vi "Pause.vi"(8 "error in (no error)":errorcluster, 11 "Pause-Resume":refnum<vi>) -> (0 "error out":errorcluster)   [LabVIEW 2014]
panel:
  # "LICENSED MATERIALS – PROPERTY OF IBM\nCopyright IBM Corp. 2016,\nALL RIGHTS RESERVED"
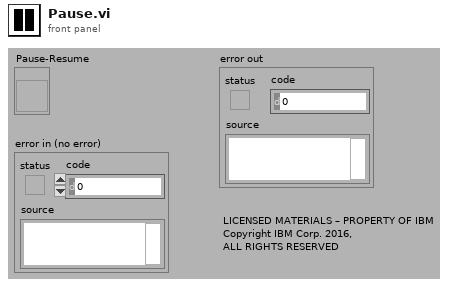
[diagram p1: front panel]
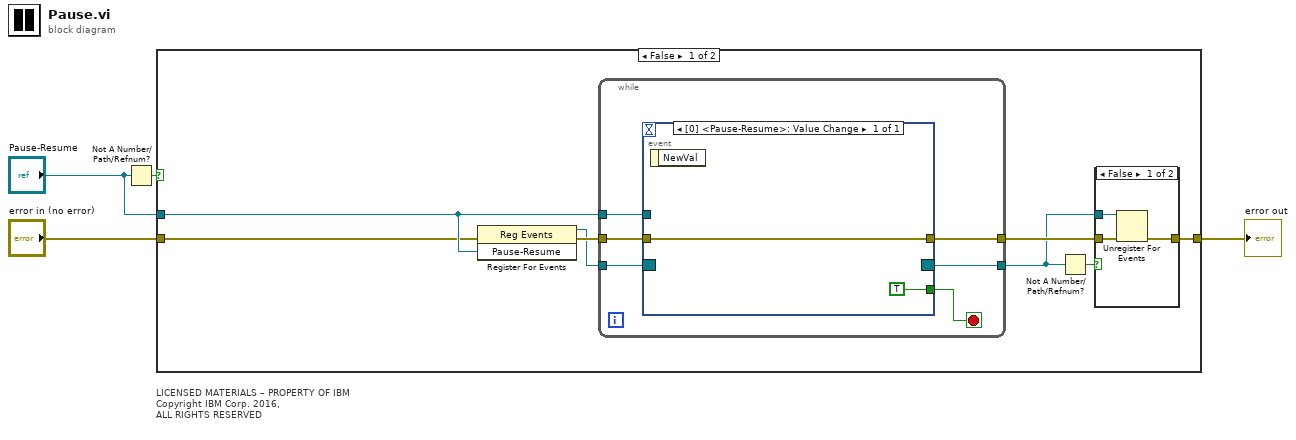
[diagram p0: block diagram]
diagram:
  # "LICENSED MATERIALS – PROPERTY OF IBM\nCopyright IBM Corp. 2016,\nALL RIGHTS RESERVED"
  n1 = Not A Number/Path/Refnum?(number/path/refnum="Pause-Resume") -> (NaN/Path/Refnum?=w3:bool)
  n2 = case shown="False" w3 {
    tunnel: "error in (no error)" -> [w5 w25]
    tunnel: [w9 w25] -> w2
    tunnel: "Pause-Resume" -> [w6 _]
    frame False {
      n3 = register-events(error in=w5, w6) -> (reference out=w8:refnum<event-registration>, error out=w11:errorcluster)  [unwired: 1 in]
      n4 = while {
        tunnel: w11 -> [w22]
        tunnel: [w21] -> w10
        tunnel: w8 -> [w20]
        tunnel: [w19] -> w7
        tunnel: w6 -> [w17]
        stop <- w18 stop-if-true
        n5 = event shown="[0] <Pause-Resume>: Value Change" {
          selector: w20 -> [_]
          dyn-events: [_] -> w19
          timeout: _ -> [_]
          tunnel: w22 -> [w23]
          tunnel: [w23] -> w21
          tunnel: [TRUE] -> w18
          tunnel: w17 -> [_]
          event Value Change {
            n6 = event-data() -> ()  [unwired: 2 out]
          }
        }
      }
      n7 = Not A Number/Path/Refnum?(number/path/refnum=w7) -> (NaN/Path/Refnum?=w12:bool)
      n8 = case shown="False" w12 {
        tunnel: [w15 w16] -> w9
        tunnel: w10 -> [w14 w16]
        tunnel: w7 -> [w13 _]
        frame False {
          n9 = Unregister For Events(event registration refnum=w13, error in=w14) -> (error out=w15:errorcluster)
        }
        frame True {
        }
      }
    }
    frame True {
    }
  }
  "error out" <- w2
